vi "setChannelArray.vi"(8 "error in (no error)":errorcluster, 10 "ChannelArray.lvclass":refnum<class "ChannelArray.lvclass">, 11 "device.lvclass in":refnum<class "device.lvclass">) -> (0 "error out":errorcluster, 3 "device.lvclass out":refnum<class "device.lvclass">)   [LabVIEW 2009, in "Tools.lvlib" / "DatabaseHelpers.lvlib" / "device.lvclass"]
uses:
  device.lvclass
  ChannelArray/ChannelArray.lvclass
  device.lvclass/device.ctl
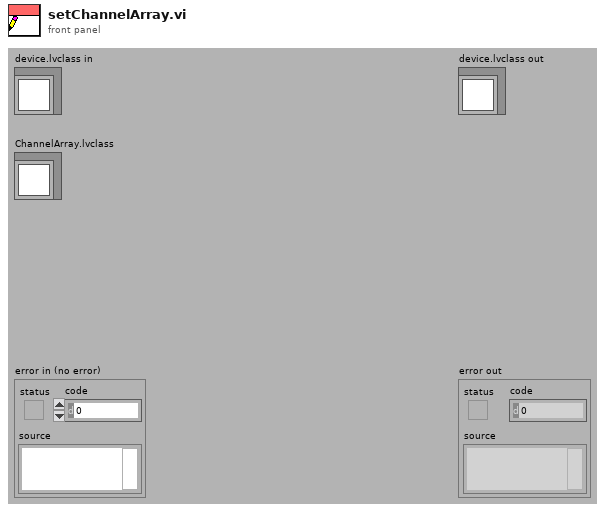
[diagram p1: front panel]
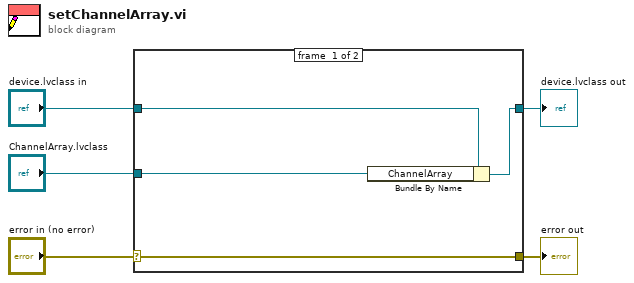
[diagram p0: block diagram]
diagram:
  n1 = case shown="No Error" "error in (no error)" {
    selector: "error in (no error)" -> [w9 w10]
    tunnel: [w9 w10] -> w4
    tunnel: [w7 w11] -> w2
    tunnel: "device.lvclass in" -> [w8 w11]
    tunnel: "ChannelArray.lvclass" -> [w6 _]
    frame #0 {
      n2 = Bundle By Name(cluster=w8, "ChannelArray"=w6) -> (w7:refnum<class "device.lvclass">)
    }
    frame #1 {
    }
  }
  "error out" <- w4
  "device.lvclass out" <- w2
